vi "LV86_Image to 32 bit arrray.vi"(2 "Flip?":bool, 3 "Image In":T1 {"Dialogs" format="%.0b"}) -> (0 "Intensity Graph":u32[][](graph), 1 "Image out":T1 {"Dialogs" format="%.0b"})   [LabVIEW 2024]
doc: "This VI converts an image into a 2-dimensional array \nof rows and columns (e.g. 320 columns and 240 rows). This is usually used for color images - where the bytes are encoded as:\n8 bits of Blue, 8 bits of Green, 8 bits of Red, and 8 bits of Greyscale to make the 32 bit integer.\n\nModifier: \nFlip: If true, this will flip the image so that the image looks right in the Intensity graph (element 0,0 in a picture is the upper left corner but in a graph is in the lower left). Default is False."
uses:
  <userlib>/ImageProcessing/QTLIB_2595_LV86/QT_Image.ctl
panel:
  # "This VI converts an image into a 2-dimensional array \nof rows and columns (e.g. 320 columns and 240 rows).  This is usually used for color images - where the bytes are encoded as:\n8 bits of Blue, 8 bits of Green, 8 bits of Red, and 8 bits of Greyscale to make the 32 bit integer.\n\nModifier: \nFlip: If true, this will flip the image so that the image looks right in the Intensity graph (element 0,0  in a picture is the upper left corner but in a graph is in the lower left). Default is False."
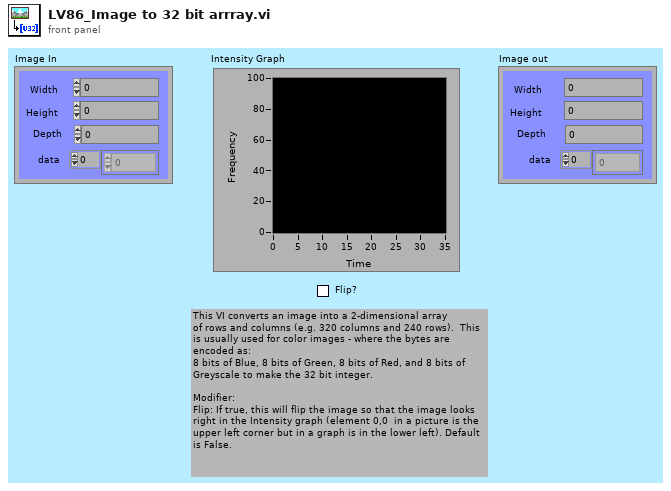
[diagram p1: front panel]
types:
  T1 = typedef "QT_Image.ctl" = cluster{"Width":i32, "Height":i32, "Depth":i32, "data":u8[], "Compressed data":u8[], "Color table":u32[], "Duration":i32, "Options":i32, "Timestamp":i32, "ID":i32, "Reserved":i32, "Dialogs":u32}
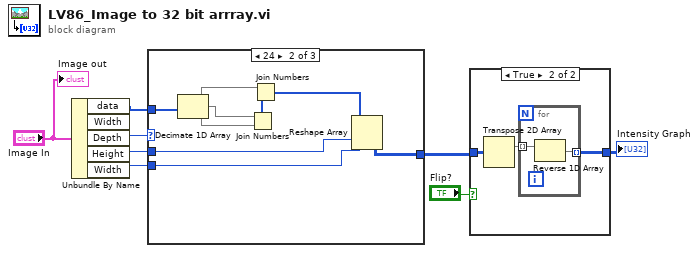
[diagram p0: block diagram]
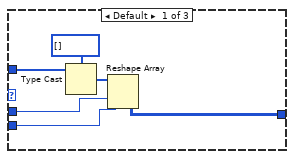
[diagram p3: hidden frame]
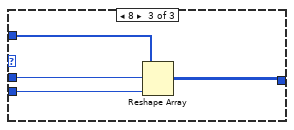
[diagram p4: hidden frame]
diagram:
  n1 = Unbundle By Name("Image In") -> ("data"=w4:u8[], "Depth"=w8:i32, "Height"=w6:i32, "Width"=w5:i32)  [unwired: 1 out]
  n2 = case shown="24" w8 {
    tunnel: w6 -> [w11 w22 w26]
    tunnel: w5 -> [w12 w23 w25]
    tunnel: [w10 w21 w24] -> w3
    tunnel: w4 -> [w9 w20 w27]
    frame Default {
      n3 = Type Cast(type=u32[] [] ("Array Constant"), x=w9) -> (*(type *) &x=w13:u32[])
      n4 = Reshape Array(w13, w11, w12) -> (w10:u32[][])
    }
    frame 24 {
      n5 = Decimate 1D Array(w20) -> (w17:u8[], w19:u8[], w18:u8[])
      n6 = Join Numbers(hi=w19, lo=w18) -> ((hi.lo)=w16:u16[])
      n7 = Join Numbers(hi=w17, lo=w16) -> ((hi.lo)=w15:u32[])
      n8 = Reshape Array(w15, w22, w23) -> (w21:u32[][])
    }
    frame 8 {
      n9 = Reshape Array(w27, w26, w25) -> (w24:u8[][])
    }
  }
  n10 = case shown="True" "Flip?" {
    tunnel: w3 -> [w28 w31]
    tunnel: [w28 w29] -> w2
    frame False {
    }
    frame True {
      n11 = Transpose 2D Array(2D array=w31) -> (transposed array=w30:u32[][])
      n12 = for {
        tunnel: w30 -> [w33] mode=indexing
        tunnel: [w32] -> w29 mode=indexing
        n13 = Reverse 1D Array(array=w33) -> (reversed array=w32:u32[])
      }
    }
  }
  "Intensity Graph" <- w2
  "Image out" <- "Image In"
